vi "move PZT center.vi"(8 "error in":errorcluster, 11 "Coarse Approach in":refnum<class "Coarse Approach.lvclass">) -> (0 "error out":errorcluster, 3 "Coarse Approach out":refnum<class "Coarse Approach.lvclass">)   [LabVIEW 2020, in "Coarse Approach.lvclass"]
uses:
  Coarse Approach.lvclass
  Coarse Approach.lvclass/Coarse Approach.ctl
  PZT/PZT.lvclass
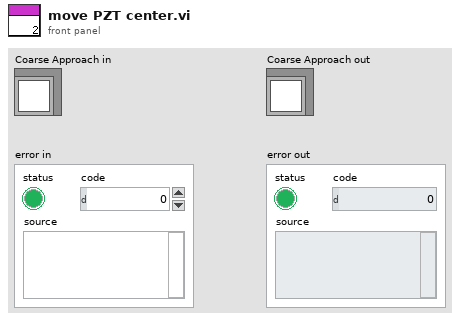
[diagram p1: front panel]
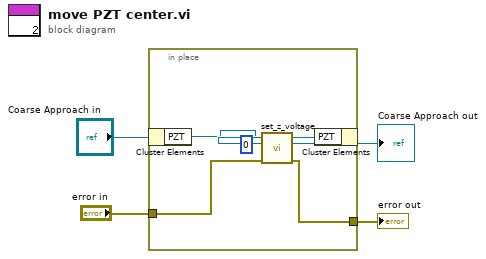
[diagram p0: block diagram]
diagram:
  n1 = in-place {
    in-place-border: "error in" -> [w7]
    in-place-border: [w9] -> w1
    n2 = in-place-cluster #1("Coarse Approach in") -> ("PZT"=w5:refnum<class "PZT.lvclass">)
    n3 = call-dynamic "set_z_voltage.vi"("error in (no error)"=w7, "Z voltage (bits)"=i16 0, "PZT in"=w5) -> ("error out"=w9:errorcluster, "PZT out"=w8:refnum<class "PZT.lvclass">)  [unwired: 7 in]
    n4 = in-place-cluster #1("PZT"=w8) -> (→"Coarse Approach out":refnum<class "Coarse Approach.lvclass">)
  }
  "error out" <- w1
